vi "Convert Database Variant to Data.vi"() -> ()   [LabVIEW 2023]
doc: "The example demonstrates how to convert database variants that you read from a database to an appropriate LabVIEW data type. For example you can convert a 1D array of database variants to a cluster of LabVIEW data. This example reads data from a predefined database, located at LabVIEW\\examples\\database\\LabVIEW.mdb, and uses the Database Variant To Data function to do the conversion. Examine the block diagram of this example VI for more information about using this function."
uses:
  <vilib>/addons/database/Connection.llb/DB Tools Open Connec (Path).vi
  <vilib>/addons/database/_DB Variant To Data/Database Variant To Data.xnode
  <vilib>/addons/database/NI_Database_API.lvlib
panel:
  out "one row":T1
  out "all data as strings":string[][](array[string])
  out "all data":T2(array[cluster])
  out "one column as strings":string[](array[string])
  # "Overview: Demonstrates the different ways to convert data with the Database Variant To Data function.\nRequirements: Database Connectivity Toolkit\nInstructions:\nRun the VI to display the same data in various formats retrieved from a database."
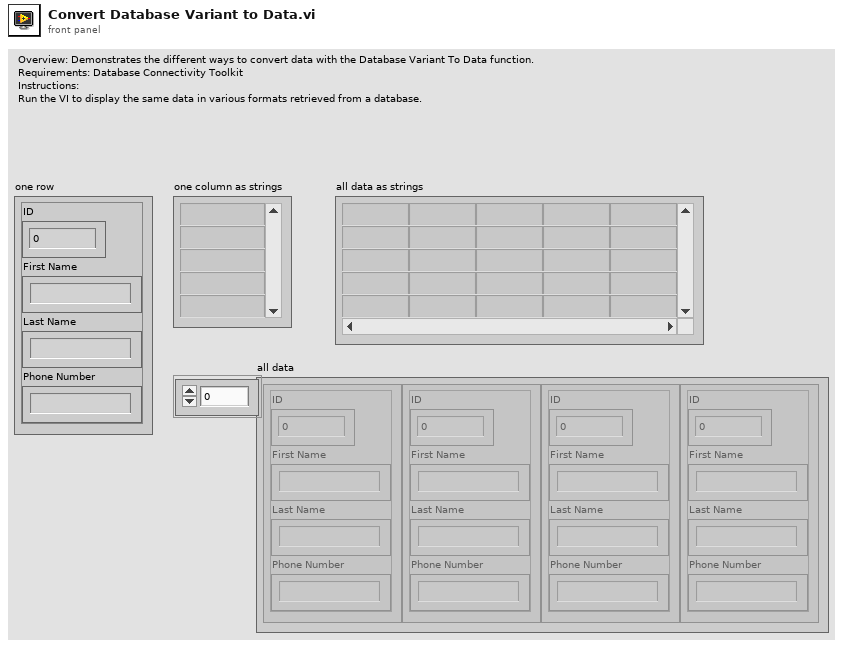
[diagram p1: front panel]
types:
  T1 = cluster{"ID":dbl, "First Name":string, "Last Name":string, "Phone Number":string}
  T2 = cluster{"ID":dbl, "First Name":string, "Last Name":string, "Phone Number":string}[]
  T3 = typedef "NI_Database_API.lvlib/Conn ObjectReference.ctl" = refnum<k1>
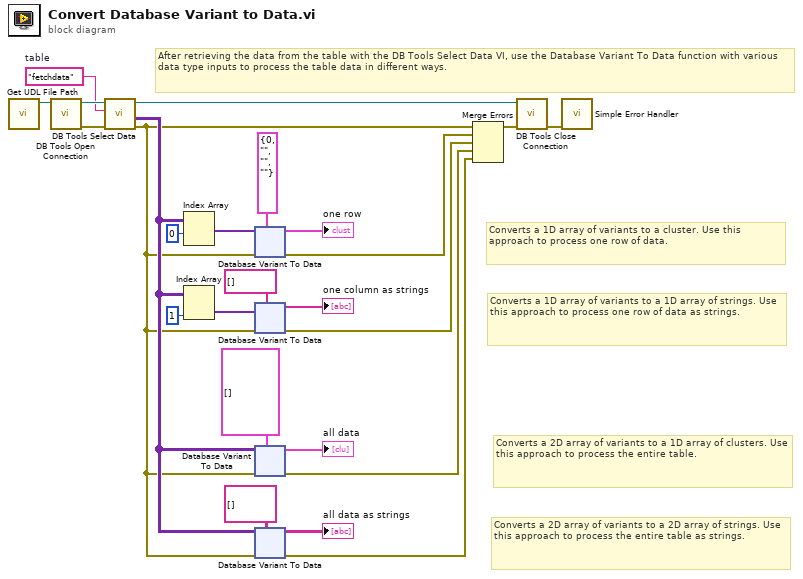
[diagram p0: block diagram]
diagram:
  w19 = "fetchdata"  # table
  # "After retrieving the data from the table with the DB Tools Select Data VI, use the Database Variant To Data function with various data type inputs to process the table data in different ways."
  # "Converts a 2D array of variants to a 2D array of strings. Use this approach to process the entire table as strings."
  # "Converts a 2D array of variants to a 1D array of clusters. Use this approach to process the entire table."
  # "Converts a 1D array of variants to a 1D array of strings. Use this approach to process one row of data as strings."
  # "Converts a 1D array of variants to a cluster. Use this approach to process one row of data."
  n1 = call "Get UDL File Path.vi"() -> ("UDL file path"=w24:path)  [unwired: 11 in]
  n2 = call-poly <vilib>:"DB Tools Open Connection.vi"("connection information"=w24) -> ("error out"=w22:errorcluster, "connection reference"=w23:T3)  [unwired: 7 in]
  n3 = call <vilib>:"DB Tools Select Data.vi"("error in (no error)"=w22, "table"=w19, "connection reference"=w23) -> ("error out"=w1:errorcluster, "data"=w3:variant[][], "connection reference out"=w21:T3)  [unwired: 3 in]
  n4 = Index Array(array=w3, index (row)=0) -> (element=w18:variant[])  [unwired: 1 in]
  n5 = Index Array(array=w3, index (col)=1 ("index (row)")) -> (element=w14:variant[])  [unwired: 1 in]
  n6 = xnode "Database Variant To Data"("database variant"=w18, "error in"=w1, "type"=cluster{i32, string, string, string} {0, "", "", ""}) -> ("data"=→"one row":cluster{i32, string, string, string}, "error out"=w20:errorcluster)
  n7 = xnode "Database Variant To Data"("database variant"=w14, "error in (no error)"=w1, "type"=string[] []) -> ("data"=→"one column as strings":string[], "error out"=w5:errorcluster)
  n8 = xnode "Database Variant To Data"("database variant"=w3, "error in (no error)"=w1, "type"=cluster{i32, string, string, string}[] []) -> ("data"=→"all data":cluster{i32, string, string, string}[], "error out"=w4:errorcluster)
  n9 = xnode "Database Variant To Data"("database variant"=w3, "error in (no error)"=w1, "type"=string[][] []) -> ("data"=→"all data as strings":string[][], "error out"=w2:errorcluster)
  n10 = Merge Errors(w1, w20, w5, w4, w2) -> (w6:errorcluster)
  n11 = call <vilib>:"DB Tools Close Connection.vi"("error in (no error)"=w6, "connection reference"=w21) -> ("error out"=w25:errorcluster)  [unwired: 5 in]
  n12 = call <vilib>:"Simple Error Handler.vi"("error in (no error)"=w25) -> ()  [unwired: 4 in, 5 out]
